vi "Main.vi"() -> ()   [LabVIEW 2019]
uses:
  <vilib>/Utility/file.llb/Write Delimited Spreadsheet (I64).vi
  <userlib>/Nanonis Prog Interface V5/Nanonis Prog Interface.lvlib
  <vilib>/ptbypt/NI_PtbyPt.lvlib
panel:
  in  "Signal index (0-127)":i8
  out "ms/loop":dbl[](array[numeric])
  out "Z position (m)":sgl format="%#_6p"
  out "Current (A)":sgl format="%#_6p"
  in  "Iterations":i32=1000
  # "Testing if Nanonis hates LabVIEW"
  # "Key:\n0: Current\n1: Z pos Read\n2: XY Move\n3: Z pos Write"
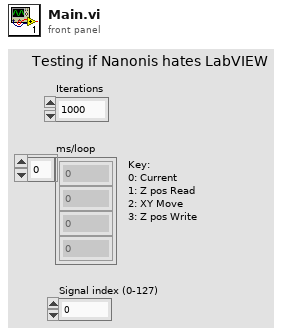
[diagram p1: front panel]
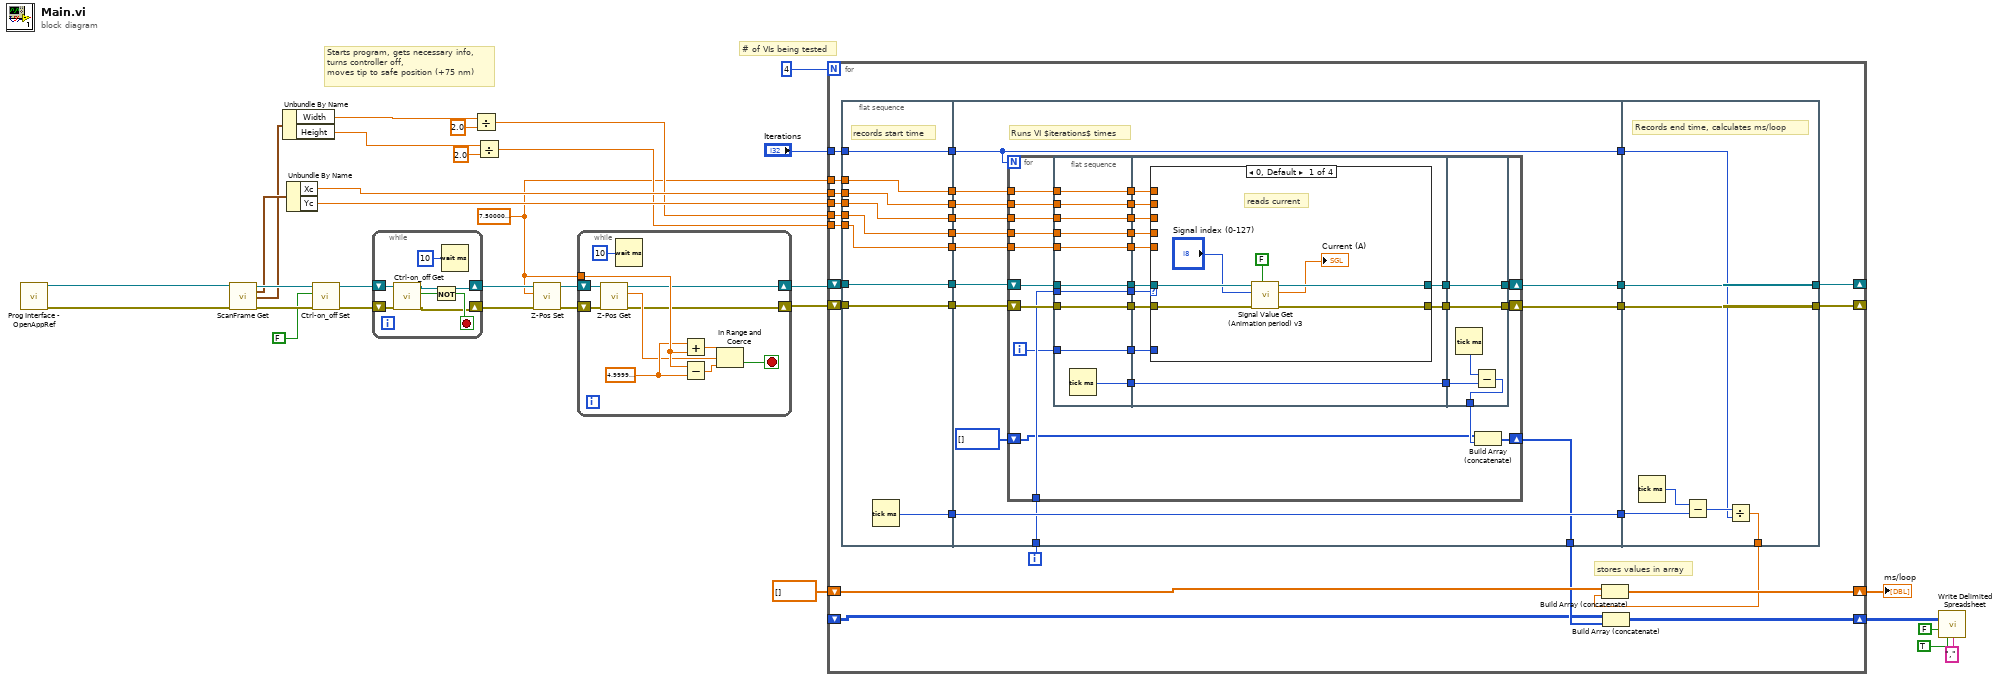
[diagram p0: block diagram]
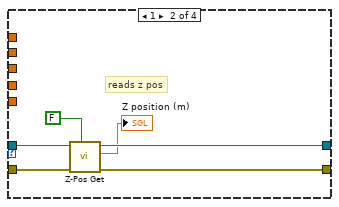
[diagram p2: hidden frame]
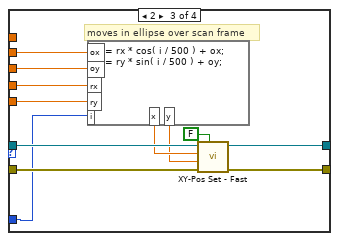
[diagram p3: hidden frame]
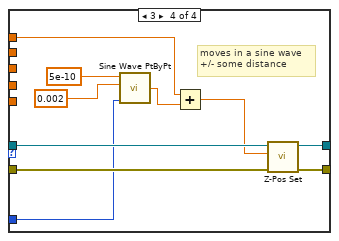
[diagram p4: hidden frame]
diagram:
  w5 = sgl 7.5e-08 ("Z position (m)")
  # "# of VIs being tested"
  # "Starts program, gets necessary info,\nturns controller off,\nmoves tip to safe position (+75 nm)"
  n1 = call <userlib>:"Prog Interface - OpenAppRef.vi"() -> ("Error out"=w28:errorcluster, "Application reference"=w29:refnum<vi>)  [unwired: 6 in]
  n2 = call <userlib>:"ScanFrame Get.vi"("Application ref in"=w29, "error in (no error)"=w28) -> ("Application ref out"=w26:refnum<vi>, "Center coordinates (m)"=w15:cluster{"Xc":sgl, "Yc":sgl}, "Size (m)"=w12:cluster{"Width":sgl, "Height":sgl}, "error out"=w25:errorcluster)  [unwired: 9 in, 1 out]
  n3 = Unbundle By Name(w12) -> ("Width"=w11:sgl, "Height"=w7:sgl)
  n4 = Unbundle By Name(w15) -> ("Xc"=w14:sgl, "Yc"=w13:sgl)
  n5 = call <userlib>:"Ctrl-on_off Set.vi"("error in (no error)"=w25, "Z Controller ON/OFF"=FALSE, "Application ref in"=w26) -> ("error out"=w22:errorcluster, "Application ref out"=w23:refnum<vi>)  [unwired: 7 in]
  n6 = while {
    shift-right: [w34] -> w21
    shift-left: w22 -> [w37]
    shift-right: [w35] -> w20
    shift-left: w23 -> [w36]
    stop <- w39 stop-if-true
    n7 = call <userlib>:"Ctrl-on_off Get.vi"("error in (no error)"=w37, "Application ref in"=w36) -> ("error out"=w34:errorcluster, "Z-Controller on/off status"=w33:bool, "Application ref out"=w35:refnum<vi>)  [unwired: 7 in]
    n8 = Not(x=w33) -> (.not. x?=w39:bool)
    n9 = Wait (ms)(milliseconds to wait=u32 10) -> ()  [unwired: 1 out]
  }
  n10 = Divide(x=w11, y=sgl 2.0) -> (x/y=w10:sgl)
  n11 = Divide(x=w7, y=sgl 2.0) -> (x/y=w6:sgl)
  n12 = call <userlib>:"Z-Pos Set.vi"("error in (no error)"=w21, "Z position (m)"=w5, "Application ref in"=w20) -> ("error out"=w18:errorcluster, "Application ref out"=w19:refnum<vi>)  [unwired: 7 in]
  n13 = while {
    shift-right: [w40] -> w16
    shift-left: w18 -> [w48]
    shift-right: [w41] -> w17
    shift-left: w19 -> [w49]
    tunnel: w5 -> [w45]
    stop <- w43 stop-if-true
    w44 = sgl 5e-10 ("x")
    n14 = call <userlib>:"Z-Pos Get.vi"("error in (no error)"=w48, "Application ref in"=w49) -> ("error out"=w40:errorcluster, "Z position (m)"=w42:sgl, "Application ref out"=w41:refnum<vi>)  [unwired: 7 in]
    n15 = Wait (ms)(milliseconds to wait=u32 10) -> ()  [unwired: 1 out]
    n16 = Add(x=w44, y=w45) -> (x+y=w47:sgl)
    n17 = Subtract(x=w45, y=w44) -> (x-y=w46:sgl)
    n18 = In Range and Coerce(upper limit=w47, x=w42, lower limit=w46) -> (In Range?=w43:bool)  [unwired: 1 out]
  }
  n19 = for {
    N: 4 -> [_]
    tunnel: "Iterations" -> [w71]
    shift-right: [w65] -> w27
    shift-left: dbl[] [] -> [w70]
    shift-right: [w69] -> _
    shift-left: w17 -> [w72]
    shift-right: [w67] -> _
    shift-left: w16 -> [w73]
    tunnel: w14 -> [w62]
    tunnel: w13 -> [w61]
    tunnel: w10 -> [w58]
    tunnel: w6 -> [w56]
    tunnel: w5 -> [w55]
    shift-right: [w52] -> w4
    shift-left: _ -> [w51]
    i -> [w74]
    # "stores values in array"
    n20 = flat-sequence {
      tunnel: [w89] -> w80
      tunnel: [w88] -> w79
      tunnel: [w87] -> w78
      tunnel: [w86] -> w77
      tunnel: w71 -> [w89]
      tunnel: w72 -> [w88]
      tunnel: w73 -> [w87]
      tunnel: [w85] -> w63
      tunnel: w62 -> [w85]
      tunnel: w61 -> [w84]
      tunnel: [w84] -> w60
      tunnel: [w83] -> w59
      tunnel: w58 -> [w83]
      tunnel: [w82] -> w57
      tunnel: w56 -> [w82]
      tunnel: w55 -> [w81]
      tunnel: [w81] -> w54
      tunnel: w80 -> [w100]
      tunnel: w79 -> [w103]
      tunnel: w78 -> [w102]
      tunnel: w77 -> [w101]
      tunnel: [w101] -> w76
      tunnel: [w100] -> w75
      tunnel: w74 -> [w99]
      tunnel: [w98] -> w68
      tunnel: [w97] -> w66
      tunnel: w63 -> [w96]
      tunnel: w60 -> [w95]
      tunnel: w59 -> [w94]
      tunnel: w57 -> [w93]
      tunnel: w54 -> [w92]
      tunnel: [w90] -> w53
      tunnel: w76 -> [w198]
      tunnel: w75 -> [w196]
      tunnel: [w195] -> w69
      tunnel: w68 -> [w195]
      tunnel: [w194] -> w67
      tunnel: w66 -> [w194]
      tunnel: [w193] -> w64
      frame #0 {
        # "records start time"
        n21 = Tick Count (ms)() -> (millisecond timer value=w86:u32)
      }
      frame #1 {
        # "Runs VI $iterations$ times"
        n22 = for {
          N: w100 -> [_]
          shift-right: [w127] -> w97
          shift-left: w102 -> [w129]
          shift-right: [w128] -> w98
          shift-left: w103 -> [w130]
          tunnel: w99 -> [w126]
          tunnel: w96 -> [w125]
          tunnel: w95 -> [w124]
          tunnel: w94 -> [w123]
          tunnel: w93 -> [w121]
          tunnel: w92 -> [w120]
          shift-right: [w105] -> w90
          shift-left: u32[] [] -> [w104]
          i -> [w122]
          n23 = flat-sequence {
            tunnel: w120 -> [w132]
            tunnel: w121 -> [w133]
            tunnel: w122 -> [w134]
            tunnel: w123 -> [w135]
            tunnel: w124 -> [w136]
            tunnel: w125 -> [w137]
            tunnel: w126 -> [w138]
            tunnel: w129 -> [w139]
            tunnel: w130 -> [w140]
            tunnel: [w140] -> w119
            tunnel: [w139] -> w118
            tunnel: [w138] -> w117
            tunnel: [w137] -> w116
            tunnel: [w136] -> w115
            tunnel: [w135] -> w114
            tunnel: [w134] -> w113
            tunnel: [w133] -> w112
            tunnel: [w132] -> w111
            tunnel: [w131] -> w108
            tunnel: w119 -> [w152]
            tunnel: w118 -> [w151]
            tunnel: w117 -> [w148]
            tunnel: w116 -> [w147]
            tunnel: w115 -> [w146]
            tunnel: w114 -> [w145]
            tunnel: w113 -> [w144]
            tunnel: w112 -> [w143]
            tunnel: w111 -> [w142]
            tunnel: [w150] -> w110
            tunnel: [w149] -> w109
            tunnel: w108 -> [w141]
            tunnel: [w141] -> w107
            tunnel: [w191] -> w127
            tunnel: [w192] -> w128
            tunnel: w110 -> [w192]
            tunnel: w109 -> [w191]
            tunnel: w107 -> [w189]
            tunnel: [w188] -> w106
            frame #0 {
              n24 = Tick Count (ms)() -> (millisecond timer value=w131:u32)
            }
            frame #1 {
              n25 = case shown="0, Default" w148 {
                tunnel: w152 -> [w159 w165 w177 w187]
                tunnel: w151 -> [w158 w164 w176 w186]
                tunnel: [w156 w162 w175 w184] -> w150
                tunnel: [w157 w163 w174 w185] -> w149
                tunnel: w147 -> [_ _ w171 _]
                tunnel: w146 -> [_ _ w170 _]
                tunnel: w145 -> [_ _ w169 _]
                tunnel: w144 -> [_ _ w168 w178]
                tunnel: w143 -> [_ _ w167 _]
                tunnel: w142 -> [_ _ _ w180]
                frame 0, Default {
                  # "reads current"
                  n26 = call <userlib>:"Signal Value Get (Animation period) v3.vi"("Wait for newest data (F=False)"=FALSE, "error in (no error)"=w158, "Signal index (0-127)"="Signal index (0-127)", "Application ref in"=w159) -> ("error out"=w157:errorcluster, "Signal value"=→"Current (A)":sgl, "Application ref out"=w156:refnum<vi>)  [unwired: 4 in]
                }
                frame 1 {
                  # "reads z pos"
                  n27 = call <userlib>:"Z-Pos Get.vi"("Wait for newest data (F=False)"=FALSE, "error in (no error)"=w164, "Application ref in"=w165) -> ("error out"=w163:errorcluster, "Z position (m)"=→"Z position (m)":sgl, "Application ref out"=w162:refnum<vi>)  [unwired: 6 in]
                }
                frame 2 {
                  # "moves in ellipse over scan frame"
                  n28 = formula code="x = rx * cos( i / 500 ) + ox;\ny = ry * sin( i / 500 ) + oy;"("rx"=w169, "i"=w168, "oy"=w170, "ox"=w171, "ry"=w167) -> ("x"=w173:dbl, "y"=w172:dbl)
                  n29 = call <userlib>:"XY-Pos Set - Fast.vi"("Wait end-of-motion (T=True)"=FALSE, "error in (no error)"=w176, "Y (m)"=w172, "X (m)"=w173, "Application ref in"=w177) -> ("error out"=w174:errorcluster, "Application ref out"=w175:refnum<vi>)  [unwired: 4 in]
                }
                frame 3 {
                  # "moves in a sine wave \n+/- some distance"
                  n30 = call <vilib>:"Sine Wave PtByPt.vi"("time"=w178, "frequency"=0.002, "amplitude"=5e-10) -> ("sine wave"=w181:dbl)  [unwired: 1 in]
                  n31 = Add(x=w180, y=w181) -> (x+y=w179:dbl)
                  n32 = call <userlib>:"Z-Pos Set.vi"("error in (no error)"=w186, "Z position (m)"=w179, "Application ref in"=w187) -> ("error out"=w185:errorcluster, "Application ref out"=w184:refnum<vi>)  [unwired: 7 in]
                }
              }
            }
            frame #2 {
              n33 = Tick Count (ms)() -> (millisecond timer value=w190:u32)
              n34 = Subtract(x=w190, y=w189) -> (x-y=w188:u32)
            }
          }
          n35 = Build Array (concatenate)(w104, w106) -> (w105:u32[])
        }
      }
      frame #2 {
        # "Records end time, calculates ms/loop"
        n36 = Tick Count (ms)() -> (millisecond timer value=w199:u32)
        n37 = Subtract(x=w199, y=w198) -> (x-y=w197:u32)
        n38 = Divide(x=w197, y=w196) -> (x/y=w193:dbl)
      }
    }
    n39 = Build Array (concatenate)(w70, w64) -> (w65:dbl[])
    n40 = Build Array (concatenate)(w51, w53) -> (w52:u32[][])
  }
  "ms/loop" <- w27
  n41 = call-poly <vilib>:"Write Delimited Spreadsheet.vi"("2D data"=w4, "append to file? (new file:F)"=FALSE, "transpose? (no:F)"=TRUE, "delimiter (\\t)"="," ("delimiter (\\t)")) -> ()  [unwired: 10 in, 2 out]
